vi "TurnToTest.vi"() -> ()   [LabVIEW 2011]
panel:
  out "New Turret Pos (Deg)":dbl
  out "Turret Pos (Deg)":dbl
  out "dx":dbl
  out "dx360":dbl
  out "AngleToTarget":dbl
  out "New Turret Pos":dbl
  in  "Turret Pos":dbl
  in  "Heading":dbl
  in  "Rx":dbl
  in  "Ry":dbl
  in  "Ty":dbl
  in  "Tx":dbl
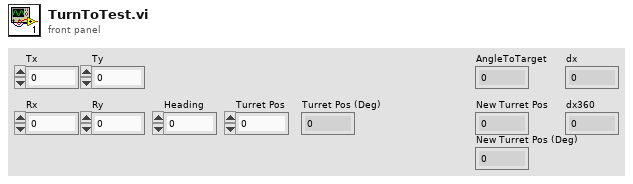
[diagram p1: front panel]
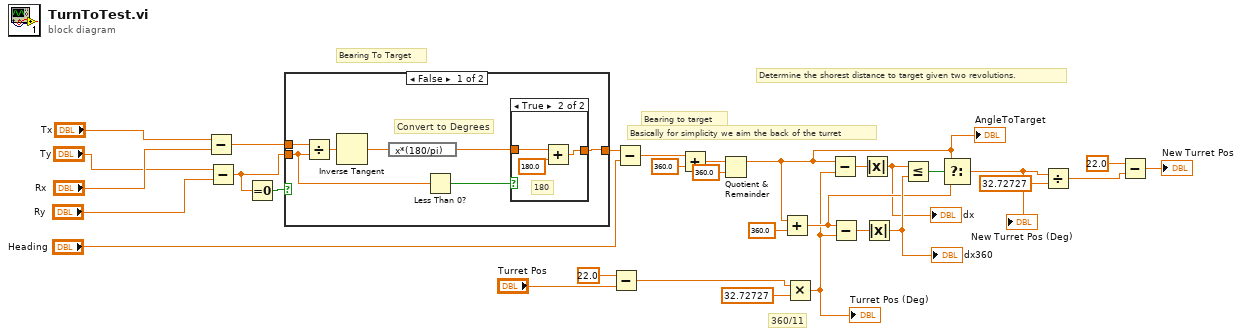
[diagram p0: block diagram]
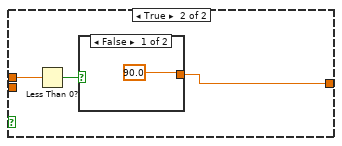
[diagram p3: hidden frame]
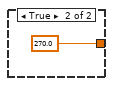
[diagram p4: hidden frame]
diagram:
  # "360/11"
  # "Bearing to target"
  # "Bearing To Target"
  # "Basically for simplicity we aim the back of the turret"
  # "Determine the shorest distance to target given two revolutions."
  n1 = Subtract(x="Tx", y="Rx") -> (x-y=w21:dbl)
  n2 = Subtract(x="Ty", y="Ry") -> (x-y=w20:dbl)
  n3 = Equal To 0?(x=w20) -> (x = 0?=w23:bool)
  n4 = case shown="False" w23 {
    tunnel: w21 -> [w38 w44]
    tunnel: [w33 w43] -> w22
    tunnel: w20 -> [w35 _]
    frame False {
      # "Convert to Degrees"
      n5 = Divide(x=w38, y=w35) -> (x/y=w36:dbl)
      n6 = Inverse Tangent(1:w36) -> (0:w37:dbl)
      n7 = expression code="x*(180/pi)"(w37) -> (w32:dbl)
      n8 = Less Than 0?(x=w35) -> (x < 0?=w34:bool)
      n9 = case shown="True" w34 {
        tunnel: [w39 w42] -> w33
        tunnel: w32 -> [w39 w41]
        frame False {
        }
        frame True {
          # "180"
          n10 = Add(x=w41, y=180.0) -> (x+y=w42:dbl)
        }
      }
    }
    frame True {
      n11 = Less Than 0?(x=w44) -> (x < 0?=w45:bool)
      n12 = case shown="False" w45 {
        tunnel: [90.0 ("y") 270.0 ("y")] -> w43
        frame False {
        }
        frame True {
        }
      }
    }
  }
  n13 = Subtract(x=22.0, y="Turret Pos") -> (x-y=w4:dbl)
  n14 = Subtract(x=w22, y="Heading") -> (x-y=w19:dbl)
  n15 = Add(x=w19, y=360.0) -> (x+y=w15:dbl)
  n16 = Quotient & Remainder(x=w15, y=360.0) -> (x-y*floor(x/y)=w18:dbl)  [unwired: 1 out]
  "AngleToTarget" <- w18
  n17 = Add(x=w18, y=360.0) -> (x+y=w25:dbl)
  n18 = Multiply(x=w4, y=32.72727) -> (x*y=w16:dbl)
  "Turret Pos (Deg)" <- w16
  n19 = Subtract(x=w18, y=w16) -> (x-y=w29:dbl)
  n20 = Subtract(x=w25, y=w16) -> (x-y=w28:dbl)
  n21 = Absolute Value(x=w29) -> (abs(x)=w7:dbl)
  "dx" <- w7
  n22 = Absolute Value(x=w28) -> (abs(x)=w27:dbl)
  "dx360" <- w27
  n23 = Less Or Equal?(x=w7, y=w27) -> (x <= y?=w26:bool)
  n24 = Select(t=w18, s=w26, f=w25) -> (s? t:f=w24:dbl)
  "New Turret Pos (Deg)" <- w24
  n25 = Divide(x=w24, y=32.72727) -> (x/y=w2:dbl)
  n26 = Subtract(x=22.0, y=w2) -> (x-y=→"New Turret Pos":dbl)
